vi "MyClient_consumer.vi"(8 "error in (no error)":errorcluster, 11 "Stop event":refnum<user-event>) -> (0 "error client":errorcluster)   [LabVIEW 2018]
uses:
  Control Packets/CONNACK/Connect Return Code -- enum.ctl
  Client/Client.lvclass/Client.ctl
  Client/Client.lvclass
  C:/Users/jdeboeck/Source/Repos/LV-MQTT-Broker/source/MQTT_Base/MQTT_Base.lvclass
  Control Packets/PUBLISH/PUBLISH.lvclass
  MQTT_Base/MQTT_Base.lvclass
  Control Packets/CONNACK/CONNACK.lvclass
panel:
  out "Random 2":dbl(graph)
  out "received":i32
  out "received timer":u32
  out "Client Status":T1=enum."Server Unavailable"
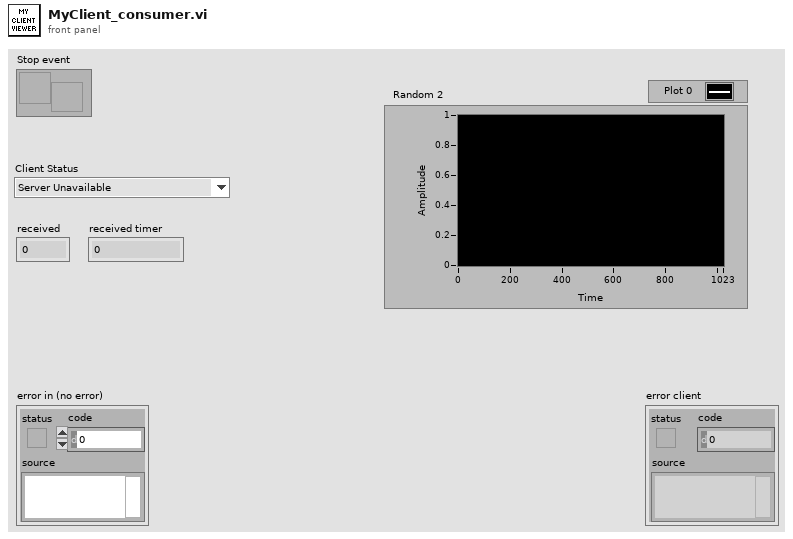
[diagram p1: front panel]
types:
  T1 = typedef "CONNACK.lvclass/Connect Return Code -- enum.ctl" = enum16{"Connection accepted", "Unacceptable protocol version", "Identifier Rejected", "Server Unavailable", "Bad Username or Password", "Not Authorized"}
  T2 = typedef "MQTT Server.lvlib/Client.lvclass/Public Events -- cluster.ctl" = cluster{"Connection Status":refnum<user-event>, "Connected":refnum<user-event>, "Application Message":refnum<user-event>}
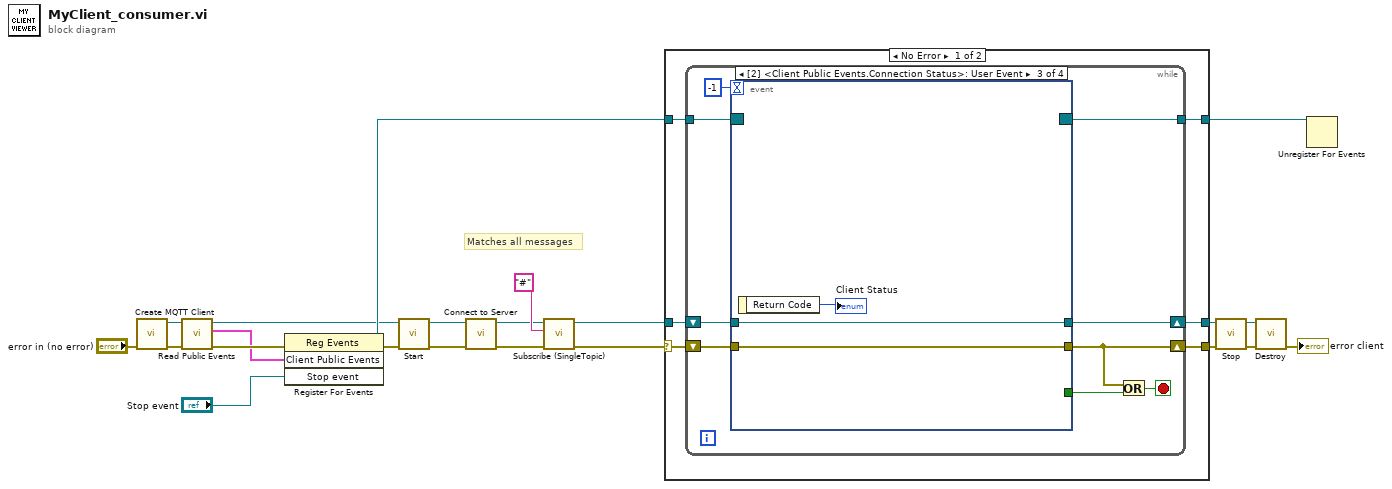
[diagram p0: block diagram]
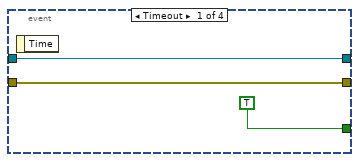
[diagram p2: hidden frame]
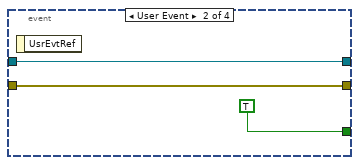
[diagram p3: hidden frame]
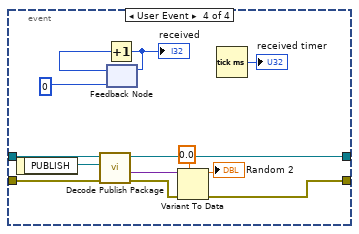
[diagram p4: hidden frame]
diagram:
  # "Matches all messages"
  n1 = call "Create MQTT Client.vi"("error in (no error)"="error in (no error)") -> ("error out"=w6:errorcluster, "Client out"=w5:refnum<class "Client.lvclass">)  [unwired: 9 in]
  n2 = call "Read Public Events.vi"("error in (no error)"=w6, "Client in"=w5) -> ("error out"=w16:errorcluster, "Client Public Events"=w15:T2, "Client out"=w7:refnum<class "Client.lvclass">)  [unwired: 7 in]
  n3 = register-events(error in=w16, w15, "Stop event") -> (reference out=w18:refnum<event-registration>, error out=w17:errorcluster)  [unwired: 1 in]
  n4 = call "Start.vi"("error in (no error)"=w17, "MQTT_Base in"=w7) -> ("error out"=w9:errorcluster, "MQTT_Base out"=w8:refnum<class "Client.lvclass">)  [unwired: 7 in, 1 out]
  n5 = call "Connect to Server.vi"("error in (no error)"=w9, "Client in"=w8) -> ("error out"=w13:errorcluster, "Client out"=w12:refnum<class "Client.lvclass">)  [unwired: 6 in, 2 out]
  n6 = call "Subscribe (SingleTopic).vi"("error in (no error)"=w13, "Topic Filter"="#", "MQTT_Base in"=w12) -> ("error out"=w3:errorcluster, "MQTT_Base out"=w20:refnum<class "Client.lvclass">)  [unwired: 7 in]
  n7 = case shown="No Error" w3 {
    selector: w3 -> [w23 w60]
    tunnel: w18 -> [w28 w62]
    tunnel: [w27 w62] -> w19
    tunnel: w20 -> [w26 w61]
    tunnel: [w25 w61] -> w21
    tunnel: [w24 w60] -> w22
    frame No Error {
      n8 = while {
        tunnel: w28 -> [w37]
        tunnel: [w36] -> w27
        shift-right: [w34] -> w25
        shift-left: w26 -> [w35]
        shift-right: [w31] -> w24
        shift-left: w23 -> [w33]
        stop <- w32 stop-if-true
        n9 = event shown="[2] <Client Public Events.Connection Status>: User Event" {
          selector: w37 -> [_ _ _ _]
          dyn-events: [_ _ _ _] -> w36
          timeout: -1 -> [_ _ _ _]
          tunnel: w35 -> [w39 w42 w45 w58]
          tunnel: [w39 w42 w45 w54] -> w34
          tunnel: [w38 w41 w44 w47] -> w31
          tunnel: w33 -> [w38 w41 w44 w53]
          tunnel: [TRUE TRUE _ _] -> w30
          event Timeout {
            n10 = event-data() -> ()  [unwired: 1 in, 1 out]
          }
          event User Event {
            n11 = event-data() -> ()  [unwired: 1 in, 1 out]
          }
          event User Event {
            n12 = event-data() -> ("Return Code"=→"Client Status":T1)  [unwired: 1 in]
          }
          event User Event {
            n13 = event-data() -> ("PUBLISH"=w59:refnum<class "PUBLISH.lvclass">)  [unwired: 1 in]
            n14 = call "Decode Publish Package.vi"("error in (no error)"=w53, "PUBLISH in"=w59, "MQTT_Base in"=w58) -> ("error out"=w48:errorcluster, "Payload"=w57:variant, "MQTT_Base out"=w54:refnum<class "Client.lvclass">)  [unwired: 5 in, 1 out]
            n15 = feedback #1(0 ("received")) -> (w51:i32)
            n16 = Increment(x=w51) -> (x+1=w50:i32)
            "received" <- w50
            n17 = feedback-in #1(w50) -> ()
            n18 = Variant To Data(error in=w48, type=0.0, Variant=w57) -> (data=→"Random 2":dbl, error out=w47:errorcluster)
            n19 = Tick Count (ms)() -> (millisecond timer value=→"received timer":u32)
          }
        }
        n20 = Or(x=w31, y=w30) -> (x .or. y?=w32:bool)
      }
    }
    frame Error {
    }
  }
  n21 = call "Stop.vi"("error in (no error)"=w22, "MQTT_Base in"=w21) -> ("error out"=w10:errorcluster, "MQTT_Base out"=w11:refnum<class "Client.lvclass">)  [unwired: 7 in, 1 out]
  n22 = call "Destroy.vi"("error in (no error)"=w10, "MQTT_Base in"=w11) -> ("error out"=→"error client":errorcluster)  [unwired: 8 in, 1 out]
  n23 = Unregister For Events(event registration refnum=w19) -> ()  [unwired: 1 in, 1 out]
